vi "testV10-AlmostDone.vi"() -> ()   [LabVIEW 2020]
uses:
  <vilib>/DAQmx/read.llb/DAQmx Read (Analog 2D DBL NChan NSamp).vi
  <vilib>/Analysis/baseanly.llb/Mean (DBL).vi
  <vilib>/DAQmx/miscellaneous.llb/DAQmx Fill In Error Info.vi
  <vilib>/Analysis/NI_AALBase.lvlib
  <resource>/objmgr/daqmx.rc
panel:
  out "index of Module 3":i32
  out "index of Module 2":i32
  out "double precision float":dbl
  out "Time Stamp":timestamp=timestamp(-21600 s since 1904-01-01)
  out "subarray 2":string[](array[string])
  out "index of Module 1":i32
  out "subarray":string[](array[string])
  in  "Counter":dbl
  out ".not. (x .or. y)?":bool
  out "index of element":i32
  out "element":dbl
  out "?":timestamp
  out "Channels":refnum<k21>[](array[refnum])
  out "size(s)":i32
  out "NumDevices":u32
  out "x/y":dbl
  in  "?":T1(tab)
  out "Sampling Status":bool
  in  "Sampling Time":u32=5
  in  "Read Time (s)":u32=60
  in  "Channel List":string(combo)="Temperature"
  out "Read Count Daily":string="0" caption="Timestamp"
  out "Countdown to Read":string="0\n 6:17:48 PM" caption="Timestamp"
  out "?":string="Timestamp"
  out "?":string="File Location"
  out "Timestamp":string="7/26/2020\n 6:17:48 PM"
  in  "Start":bool
  in  "Next Button":bool
  in  "Stop Button 2":bool
  out "Graph Running":bool
  in  "Resolution":u8=10 min=10
  in  "Stop Button":bool
  in  "Play Button":bool
  out "Module 3":bool
  out "Module 2":bool
  out "Module 1":bool
  out "3":bool
  out "2":bool
  out "1":bool
  in  "Running Module":u8=1 min=1 max=3
  in  "Module 3 Task":refnum<k21>="MyTemperatureTask_2"
  out "?":waveform(dbl)(graph)
  in  "Module 3 File Data Location":path=path "E:/KMUTT/Master Degree/labviewjgsee/log/Module3"
  in  "Module 2 File Data Location":path=path "E:/KMUTT/Master Degree/labviewjgsee/log/Module2"
  in  "Module 2 Task":refnum<k21>="MyTemperatureTask_1"
  in  "Module 1 File Data Location":path=path "E:/KMUTT/Master Degree/labviewjgsee/log/Module1"
  in  "Module 1 Task":refnum<k21>="MyTemperatureTask"
  in  "DAQmx Device Name":tag="JGSEE"
  out "Table Module 1":string[][](table)
  out "Table Module 2":string[][](table)
  out "Table Module 3":string[][](table)
  in  "Select Channel Module 1":string(combo)
  out "?":string="Date"
  out "Timestamp 2":string="7/26/2020\n 6:17:48 PM" caption="Timestamp"
  out "Graph Module 1":cluster{timestamp[], dbl[]}[](graph)
  in  "Select Channel Module 2":string(combo)
  out "?":string="Date"
  out "Timestamp 3":string="7/26/2020\n 6:17:48 PM" caption="Timestamp"
  out "Graph Module 2":cluster{timestamp[], dbl[]}[](graph)
  in  "Select Channel Module 3":string(combo)
  out "?":string="Date"
  out "Timestamp 4":string="7/26/2020\n 6:17:48 PM" caption="Timestamp"
  out "Graph Module 3":cluster{timestamp[], dbl[]}[](graph)
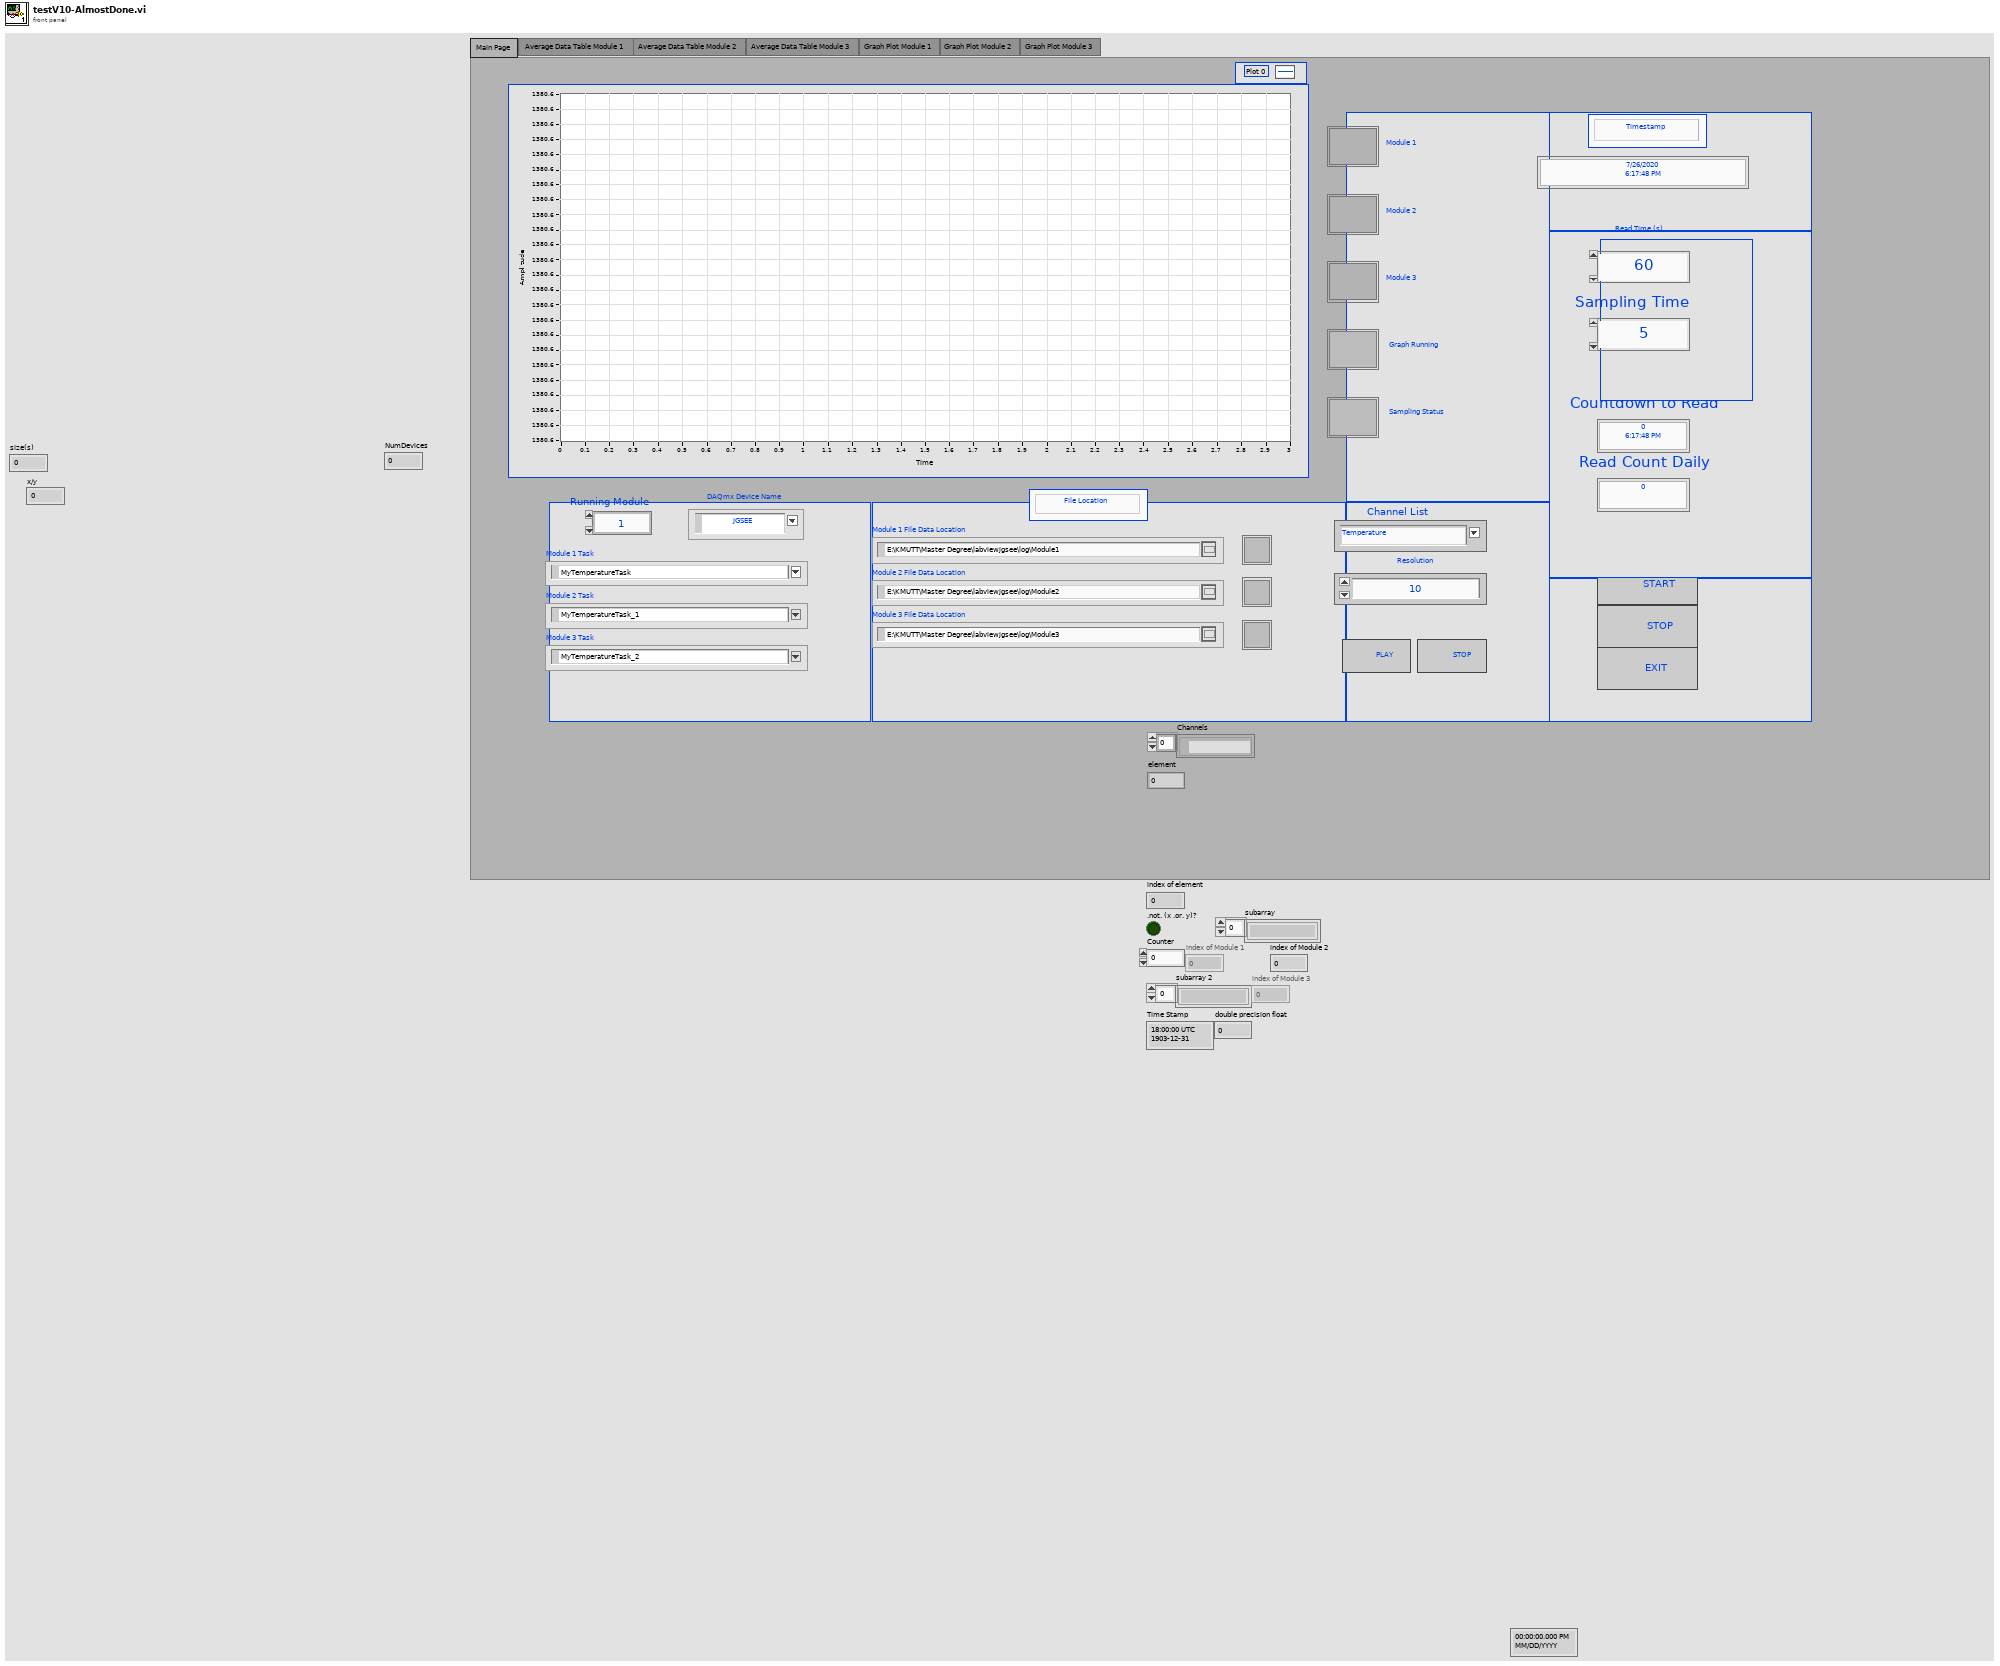
[diagram p1: front panel]
types:
  T1 = enum32{"Main Page ", " Average Data Table Module 1", "Average Data Table Module 2", "Average Data Table Module 3", "Graph Plot Module 1", "Graph Plot Module 2", "Graph Plot Module 3"}
  T2 = enum16{"open", "replace", "create", "open or create", "replace or create", "replace or create with confirmation"}
  T3 = enum8{"Enabled", "Disabled", "Disabled and Grayed Out"}
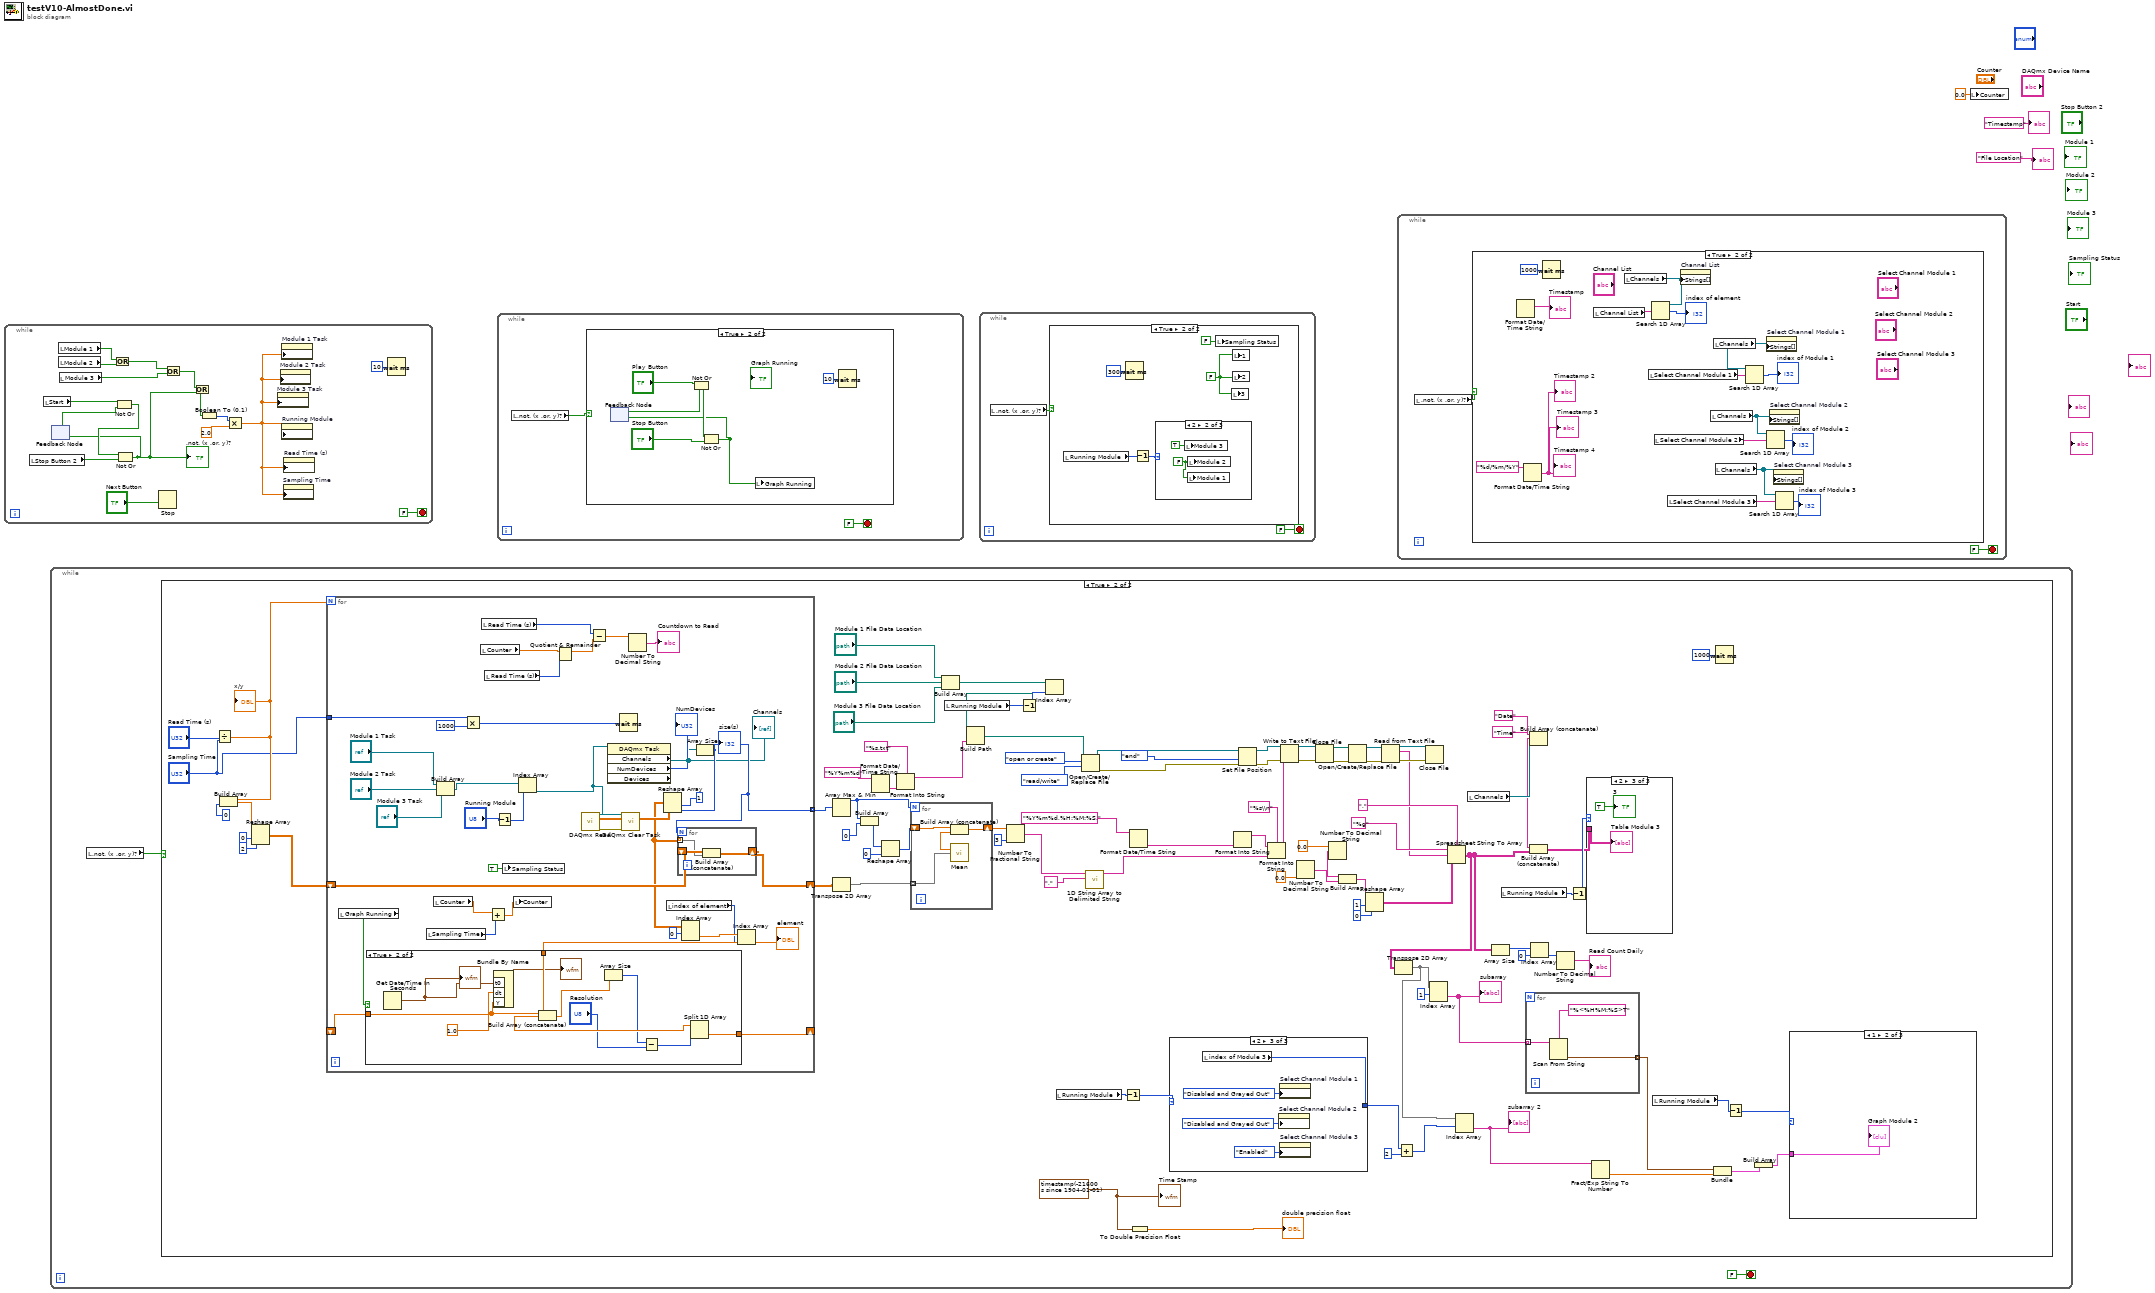
[diagram p0: block diagram]
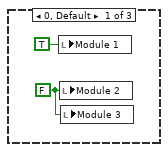
[diagram p4: hidden frame]
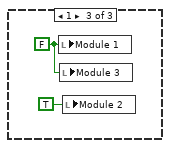
[diagram p5: hidden frame]
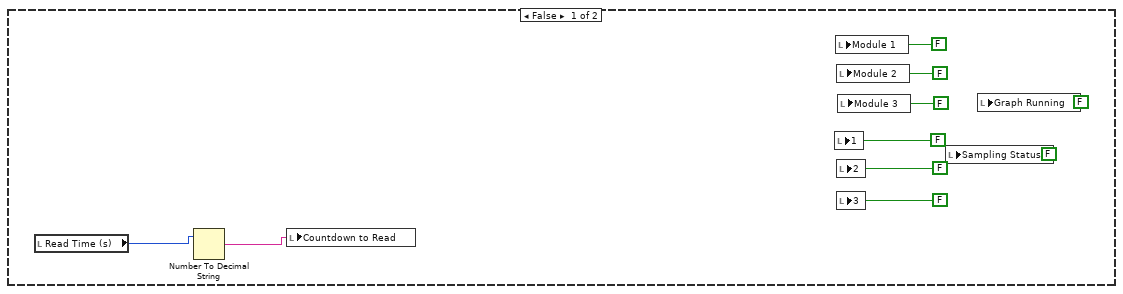
[diagram p7: hidden frame]
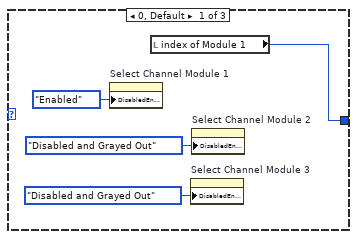
[diagram p8: hidden frame]
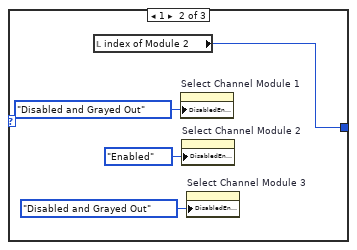
[diagram p9: hidden frame]
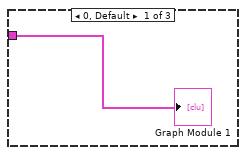
[diagram p10: hidden frame]
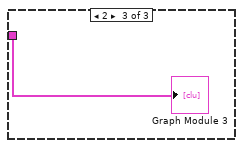
[diagram p11: hidden frame]
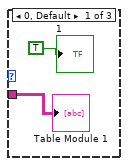
[diagram p12: hidden frame]
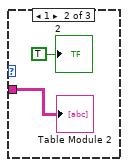
[diagram p13: hidden frame]
diagram:
  n1 = while {
    stop <- FALSE stop-if-true
    n2 = local read "Stop Button 2"() -> (w19:bool)
    n3 = local read "Start"() -> (w14:bool)
    n4 = feedback #1() -> (w17:bool)  [unwired: 1 in]
    n5 = local read "Module 1"() -> (w12:bool)
    n6 = local read "Module 2"() -> (w11:bool)
    n7 = local read "Module 3"() -> (w9:bool)
    n8 = Or(x=w12, y=w11) -> (x .or. y?=w10:bool)
    n9 = Not Or(1:w17, 2:w14) -> (0:w18:bool)
    n10 = Not Or(1:w19, 2:w18) -> (0:w6:bool)
    ".not. (x .or. y)?" <- w6
    n11 = feedback-in #1(w6) -> ()
    n12 = Stop(stop? (T)="Next Button") -> ()
    n13 = Or(x=w10, y=w9) -> (x .or. y?=w8:bool)
    n14 = Or(x=w8, y=w6) -> (x .or. y?=w5:bool)
    n15 = Boolean To (0,1)(Boolean=w5) -> (0, 1=w7:i16)
    n16 = Multiply(x=w7, y=2.0) -> (x*y=w4:dbl)
    n17 = property on="Module 3 Task" class="DAQmxName (strict)"("DisabledEnum"=w4) -> ()  [unwired: 2 in, 2 out]
    n18 = property on="Module 2 Task" class="DAQmxName (strict)"("DisabledEnum"=w4) -> ()  [unwired: 2 in, 2 out]
    n19 = property on="Module 1 Task" class="DAQmxName (strict)"("DisabledEnum"=w4) -> ()  [unwired: 2 in, 2 out]
    n20 = property on="Running Module" class="DigNum (strict)"("DisabledEnum"=w4) -> ()  [unwired: 2 in, 2 out]
    n21 = property on="Sampling Time" class="DigNum (strict)"("DisabledEnum"=w4) -> ()  [unwired: 2 in, 2 out]
    n22 = property on="Read Time (s)" class="DigNum (strict)"("DisabledEnum"=w4) -> ()  [unwired: 2 in, 2 out]
    n23 = Wait (ms)(milliseconds to wait=u32 10) -> ()  [unwired: 1 out]
  }
  n24 = while {
    stop <- FALSE stop-if-true
    n25 = local read ".not. (x .or. y)?"() -> (w21:bool)
    n26 = case shown="True" w21 {
      frame False {
        n27 = local read "Read Time (s)"() -> (w24:u32)
        n28 = Number To Decimal String(number=w24) -> (decimal integer string=w23:string)  [unwired: 1 in]
        n29 = local write "Countdown to Read"(w23) -> ()
        n30 = local write "1"(FALSE ("1")) -> ()
        n31 = local write "Module 1"(FALSE ("Module 1")) -> ()
        n32 = local write "Module 2"(FALSE ("Module 2")) -> ()
        n33 = local write "2"(FALSE ("2")) -> ()
        n34 = local write "3"(FALSE ("3")) -> ()
        n35 = local write "Module 3"(FALSE ("Module 3")) -> ()
        n36 = local write "Sampling Status"(FALSE ("Sampling Status")) -> ()
        n37 = local write "Graph Running"(FALSE ("Graph Running")) -> ()
      }
      frame True {
        w40 = timestamp(-21600 s since 1904-01-01)
        n38 = Divide(x="Read Time (s)", y="Sampling Time") -> (x/y=w102:dbl)
        "x/y" <- w102
        n39 = Build Array(w102, 0 ("element")) -> (w106:dbl[])
        n40 = Reshape Array(w106, 0 ("dimension size"), 2 ("dimension size")) -> (w103:dbl[][])
        n41 = for {
          N: w102 -> [_]
          shift-right: [w184] -> w71
          shift-left: w103 -> [w183]
          tunnel: "Sampling Time" -> [w182]
          tunnel: [w180] -> w101 mode=indexing
          shift-right: [w164] -> _
          shift-left: _ -> [w163]
          n42 = local read "Graph Running"() -> (w162:bool)
          n43 = local read "Sampling Time"() -> (w158:u32)
          n44 = local read "Counter"() -> (w157:dbl)
          n45 = Build Array("Module 1 Task", "Module 2 Task", "Module 3 Task") -> (w175:refnum<k21>[])
          n46 = Multiply(x=w182, y=u32 1000) -> (x*y=w170:u32)
          n47 = local read "Counter"() -> (w151:dbl)
          n48 = local read "Read Time (s)"() -> (w154:u32)
          n49 = local read "Read Time (s)"() -> (w156:u32)
          n50 = Add(x=w157, y=w158) -> (x+y=w159:dbl)
          n51 = Decrement(x="Running Module") -> (x-1=w171:u8)
          n52 = local write "Sampling Status"(TRUE ("Sampling Status")) -> ()
          n53 = local write "Counter"(w159) -> ()
          n54 = Index Array(array=w175, index=w171) -> (element=w174:refnum<k21>)
          n55 = Quotient & Remainder(x=w151, y=w156) -> (x-y*floor(x/y)=w155:dbl)  [unwired: 1 out]
          n56 = call-poly <vilib>:"DAQmx Read.vi"("task/channels in"=w174) -> ("task out"=w186:refnum<k21>, "data"=w179:dbl[][], "error out"=w187:errorcluster)  [unwired: 12 in]
          n57 = Subtract(x=w154, y=w155) -> (x-y=w153:dbl)
          n58 = property class="DAQmx Task" props=["Channels", "NumDevices", "Devices"](reference=w174) -> ("Channels"=w169:refnum<k21>[], "NumDevices"=→"NumDevices":u32)  [unwired: 1 in, 3 out]
          "Channels" <- w169
          n59 = Wait (ms)(milliseconds to wait=w170) -> ()  [unwired: 1 out]
          n60 = call <vilib>:"DAQmx Clear Task.vi"("task in"=w186, "error in"=w187) -> ()  [unwired: 13 in, 1 out]
          n61 = Number To Decimal String(number=w153) -> (decimal integer string=→"Countdown to Read":string)  [unwired: 1 in]
          n62 = local read "index of element"() -> (w161:i32)
          n63 = Array Size(array=w169) -> (size(s)=w180:i32)
          "size(s)" <- w180
          n64 = Reshape Array(w179, 1 ("dimension size"), w180) -> (w168:dbl[][])
          n65 = for {
            N: w180 -> [_]
            shift-right: [w199] -> w184
            shift-left: w183 -> [w200]
            tunnel: w168 -> [w198] mode=indexing
            n66 = Build Array (concatenate)(w200, w198) -> (w199:dbl[][])
          }
          n67 = Index Array(array=w168, index (row)=0) -> (element=w166:dbl[])  [unwired: 1 in]
          n68 = Index Array(array=w166, index=w161) -> (element=w165:dbl)
          "element" <- w165
          n69 = case shown="True" w162 {
            tunnel: w165 -> [_ w195]
            tunnel: [_ w192] -> w164
            tunnel: w163 -> [_ w191]
            frame False {
            }
            frame True {
              n70 = Get Date/Time In Seconds() -> (seconds since 1Jan1904=w197:timestamp)
              "?" <- w197
              n71 = Bundle By Name("t0"=w197, "dt"=1.0, "Y"=w191) -> (→"?":waveform(dbl))  [unwired: 1 in]
              n72 = Build Array (concatenate)(w191, w195) -> (w193:dbl[])
              n73 = Array Size(array=w193) -> (size(s)=w189:i32)
              n74 = Subtract(x=w189, y="Resolution") -> (x-y=w190:i32)
              n75 = Split 1D Array(array=w193, index=w190) -> (second subarray=w192:dbl[])  [unwired: 1 out]
            }
          }
        }
        n76 = Array Max & Min(array=w101) -> (max value=w98:i32)  [unwired: 3 out]
        n77 = Transpose 2D Array(2D array=w71) -> (transposed array=w100:dbl[][])
        n78 = Build Array(w98, 0 ("element")) -> (w96:i32[])
        n79 = Format Date/Time String(time format string (%c)="%Y%m%d") -> (date/time string=w118:string)  [unwired: 2 in]
        n80 = Reshape Array(w96, 0 ("dimension size")) -> (w95:i32[])
        n81 = Format Into String(format string="%s.txt", w118) -> (resulting string=w116:string)  [unwired: 2 in, 1 out]
        n82 = for {
          N: w98 -> [_]
          tunnel: w100 -> [w204] mode=indexing
          shift-right: [w202] -> w108
          shift-left: w95 -> [w201]
          n83 = call-poly <vilib>:"Mean.vi"("X"=w204) -> ("mean"=w203:dbl)  [unwired: 1 out]
          n84 = Build Array (concatenate)(w201, w203) -> (w202:dbl[])
        }
        n85 = Build Array("Module 1 File Data Location", "Module 2 File Data Location", "Module 3 File Data Location") -> (w64:path[])
        n86 = local read "Running Module"() -> (w65:u8)
        n87 = Number To Fractional String(number=w108, precision (6)=i16 3) -> (F-format string=w109:string[])  [unwired: 2 in]
        n88 = Decrement(x=w65) -> (x-1=w63:u8)
        n89 = Index Array(array=w64, index=w63) -> (element=w62:path)
        n90 = Build Path(base path=w62, name or relative path=w116) -> (appended path=w115:path)
        n91 = local read "Running Module"() -> (w38:u8)
        n92 = Open/Create/Replace File(file path (use dialog)=w115, operation (0:open)=T2."open or create", access (0:read/write)=enum16{"read/write", "read-only", "write-only"}."read/write") -> (refnum out=w93:refnum<file>, error out=w122:errorcluster)  [unwired: 3 in, 1 out]
        n93 = call <vilib>:"1D String Array to Delimited String.vi"("delimiter"="," ("format string"), "string array"=w109) -> ("delimited string"=w114:string)  [unwired: 9 in]
        n94 = Decrement(x=w38) -> (x-1=w37:u8)
        n95 = Format Date/Time String(time format string (%c)="%Y%m%d,%H:%M:%S,") -> (date/time string=w111:string)  [unwired: 2 in]
        n96 = To Double Precision Float(number=w40) -> (double precision float=→"double precision float":dbl)
        n97 = case shown="2" w37 {
          tunnel: [w130 w134 w138] -> w33
          frame 0, Default {
            n98 = property on="Select Channel Module 1" class="CmbBox"("DisabledEnum"=T3."Enabled" ("Disabled")) -> ()  [unwired: 2 in, 2 out]
            n99 = local read "index of Module 1"() -> (w130:i32)
            n100 = property on="Select Channel Module 3" class="CmbBox"("DisabledEnum"=T3."Disabled and Grayed Out" ("Disabled")) -> ()  [unwired: 2 in, 2 out]
            n101 = property on="Select Channel Module 2" class="CmbBox"("DisabledEnum"=T3."Disabled and Grayed Out" ("Disabled")) -> ()  [unwired: 2 in, 2 out]
          }
          frame 1 {
            n102 = local read "index of Module 2"() -> (w134:i32)
            n103 = property on="Select Channel Module 1" class="CmbBox"("DisabledEnum"=T3."Disabled and Grayed Out" ("Disabled")) -> ()  [unwired: 2 in, 2 out]
            n104 = property on="Select Channel Module 2" class="CmbBox"("DisabledEnum"=T3."Enabled" ("Disabled")) -> ()  [unwired: 2 in, 2 out]
            n105 = property on="Select Channel Module 3" class="CmbBox"("DisabledEnum"=T3."Disabled and Grayed Out" ("Disabled")) -> ()  [unwired: 2 in, 2 out]
          }
          frame 2 {
            n106 = local read "index of Module 3"() -> (w138:i32)
            n107 = property on="Select Channel Module 2" class="CmbBox"("DisabledEnum"=T3."Disabled and Grayed Out" ("Disabled")) -> ()  [unwired: 2 in, 2 out]
            n108 = property on="Select Channel Module 1" class="CmbBox"("DisabledEnum"=T3."Disabled and Grayed Out" ("Disabled")) -> ()  [unwired: 2 in, 2 out]
            n109 = property on="Select Channel Module 3" class="CmbBox"("DisabledEnum"=T3."Enabled" ("Disabled")) -> ()  [unwired: 2 in, 2 out]
          }
        }
        n110 = Format Into String(w111) -> (resulting string=w110:string)  [unwired: 3 in, 1 out]
        n111 = Set File Position(refnum=w93, from (0:start)=enum16{"start", "end", "current"}."end", error in=w122) -> (refnum out=w123:refnum<file>, error out=w121:errorcluster)  [unwired: 1 in]
        n112 = Format Into String(format string="%s\\n", initial string=w110, w114) -> (resulting string=w85:string)  [unwired: 1 in, 1 out]
        n113 = Write to Text File(file (use dialog)=w123, text=w85, error in=w121) -> (refnum out=w92:refnum<file>, error out=w91:errorcluster)  [unwired: 1 in, 1 out]
        n114 = Number To Decimal String(number=0.0 ("element")) -> (decimal integer string=w73:string)  [unwired: 1 in]
        n115 = Close File(refnum=w92, error in=w91) -> (path=w90:path, error out=w89:errorcluster)
        n116 = Number To Decimal String(number=0.0 ("element")) -> (decimal integer string=w75:string)  [unwired: 1 in]
        n117 = Build Array(w75, w73) -> (w77:string[])
        n118 = Open/Create/Replace File(file path (use dialog)=w90, error in=w89) -> (refnum out=w88:refnum<file>, error out=w87:errorcluster)  [unwired: 4 in, 1 out]
        n119 = Reshape Array(w77, 1 ("dimension size"), 0 ("dimension size")) -> (w78:string[][])
        n120 = Read from Text File(file (use dialog)=w88, error in=w87) -> (refnum out=w86:refnum<file>, text=w81:string, error out=w82:errorcluster)  [unwired: 2 in, 1 out]
        n121 = Add(x=w33, y=2) -> (x+y=w46:i32)
        n122 = Close File(refnum=w86, error in=w82) -> ()  [unwired: 2 out]
        n123 = Spreadsheet String To Array(delimiter (Tab)=",", format string="%g", spreadsheet string=w81, array type (2D Dbl)=w78) -> (array=w50:string[][])
        n124 = Transpose 2D Array(2D array=w50) -> (transposed array=w47:string[][])
        n125 = Index Array(array=w47, index (row)=1 ("index")) -> (element=w45:string[])  [unwired: 1 in]
        "subarray" <- w45
        n126 = Index Array(array=w47, index (row)=w46) -> (element=w43:string[])  [unwired: 1 in]
        "subarray 2" <- w43
        n127 = local read "Channels"() -> (w56:refnum<k21>[])
        n128 = Array Size(array=w50) -> (size(s)=w54:i32[])
        n129 = local read "Running Module"() -> (w61:u8)
        n130 = for {
          tunnel: w45 -> [w143] mode=indexing
          tunnel: [w142] -> w41 mode=indexing
          n131 = Scan From String(format string="%<%H%M:%S>T", input string=w143) -> (output 1=w142:timestamp)  [unwired: 3 in, 3 out]
        }
        n132 = Build Array (concatenate)("Date", "Time", w56) -> (w55:string[])
        n133 = Build Array (concatenate)(w55, w50) -> (w59:string[][])
        n134 = Index Array(array=w54, index=0) -> (element=w52:i32)
        n135 = Number To Decimal String(number=w52) -> (decimal integer string=→"Read Count Daily":string)  [unwired: 1 in]
        n136 = Decrement(x=w61) -> (x-1=w60:u8)
        n137 = case shown="2" w60 {
          tunnel: w59 -> [w146 w148 w150]
          frame 0, Default {
            "Table Module 1" <- w146
            "1" <- TRUE ("1")
          }
          frame 1 {
            "Table Module 2" <- w148
            "2" <- TRUE ("2")
          }
          frame 2 {
            "Table Module 3" <- w150
            "3" <- TRUE ("3")
          }
        }
        n138 = Fract/Exp String To Number(string=w43) -> (number=w42:dbl[])  [unwired: 3 in, 1 out]
        n139 = local read "Running Module"() -> (w36:u8)
        n140 = Bundle(w41, w42) -> (w44:cluster{timestamp[], dbl[]})  [unwired: 1 in]
        n141 = Wait (ms)(milliseconds to wait=u32 1000) -> ()  [unwired: 1 out]
        n142 = Decrement(x=w36) -> (x-1=w35:u8)
        n143 = Build Array(w44) -> (w34:cluster{timestamp[], dbl[]}[])
        n144 = case shown="1" w35 {
          tunnel: w34 -> [w139 w140 w141]
          frame 0, Default {
            "Graph Module 1" <- w139
          }
          frame 1 {
            "Graph Module 2" <- w140
          }
          frame 2 {
            "Graph Module 3" <- w141
          }
        }
        "Time Stamp" <- w40
      }
    }
  }
  n145 = while {
    stop <- FALSE stop-if-true
    n146 = local read ".not. (x .or. y)?"() -> (w205:bool)
    n147 = case shown="True" w205 {
      frame False {
      }
      frame True {
        n148 = feedback #2() -> (w208:bool)  [unwired: 1 in]
        n149 = Not Or(1:w208, 2:"Play Button") -> (0:w209:bool)
        n150 = Not Or(1:"Stop Button", 2:w209) -> (0:w207:bool)
        n151 = feedback-in #2(w207) -> ()
        n152 = local write "Graph Running"(w207) -> ()
        n153 = Wait (ms)(milliseconds to wait=u32 10) -> ()  [unwired: 1 out]
      }
    }
  }
  n154 = while {
    stop <- FALSE stop-if-true
    n155 = local read ".not. (x .or. y)?"() -> (w213:bool)
    n156 = case shown="True" w213 {
      frame False {
      }
      frame True {
        w218 = FALSE ("1")
        n157 = local read "Running Module"() -> (w216:u8)
        n158 = Wait (ms)(milliseconds to wait=u32 300) -> ()  [unwired: 1 out]
        n159 = Decrement(x=w216) -> (x-1=w215:u8)
        n160 = case shown="2" w215 {
          frame 0, Default {
            w221 = FALSE ("Module 2")
            n161 = local write "Module 1"(TRUE ("Module 1")) -> ()
            n162 = local write "Module 2"(w221) -> ()
            n163 = local write "Module 3"(w221) -> ()
          }
          frame 2 {
            w223 = FALSE ("Module 2")
            n164 = local write "Module 3"(TRUE ("Module 3")) -> ()
            n165 = local write "Module 1"(w223) -> ()
            n166 = local write "Module 2"(w223) -> ()
          }
          frame 1 {
            w225 = FALSE ("Module 1")
            n167 = local write "Module 1"(w225) -> ()
            n168 = local write "Module 3"(w225) -> ()
            n169 = local write "Module 2"(TRUE ("Module 2")) -> ()
          }
        }
        n170 = local write "Sampling Status"(FALSE ("Sampling Status")) -> ()
        n171 = local write "3"(w218) -> ()
        n172 = local write "1"(w218) -> ()
        n173 = local write "2"(w218) -> ()
      }
    }
  }
  n174 = while {
    stop <- FALSE stop-if-true
    n175 = local read ".not. (x .or. y)?"() -> (w226:bool)
    n176 = case shown="True" w226 {
      frame False {
      }
      frame True {
        n177 = Format Date/Time String() -> (date/time string=→"Timestamp":string)  [unwired: 3 in]
        n178 = Format Date/Time String(time format string (%c)="%d/%m/%Y") -> (date/time string=→"Timestamp 2" →"Timestamp 3" →"Timestamp 4":string)  [unwired: 2 in]
        n179 = Wait (ms)(milliseconds to wait=u32 1000) -> ()  [unwired: 1 out]
        n180 = local read "Channel List"() -> (w242:string)
        n181 = local read "Channels"() -> (w243:refnum<k21>[])
        n182 = local read "Select Channel Module 1"() -> (w238:string)
        n183 = Search 1D Array(1D array=w243, element=w242) -> (index of element=→"index of element":i32)  [unwired: 1 in]
        n184 = local read "Select Channel Module 2"() -> (w236:string)
        n185 = local read "Select Channel Module 3"() -> (w233:string)
        n186 = property on="Channel List" class="CmbBox"("Strings[]"=w243) -> ()  [unwired: 2 in, 2 out]
        n187 = local read "Channels"() -> (w235:refnum<k21>[])
        n188 = local read "Channels"() -> (w239:refnum<k21>[])
        n189 = local read "Channels"() -> (w232:refnum<k21>[])
        n190 = Search 1D Array(1D array=w239, element=w238) -> (index of element=→"index of Module 1":i32)  [unwired: 1 in]
        n191 = Search 1D Array(1D array=w235, element=w236) -> (index of element=→"index of Module 2":i32)  [unwired: 1 in]
        n192 = property on="Select Channel Module 1" class="CmbBox"("Strings[]"=w239) -> ()  [unwired: 2 in, 2 out]
        n193 = property on="Select Channel Module 2" class="CmbBox"("Strings[]"=w235) -> ()  [unwired: 2 in, 2 out]
        n194 = property on="Select Channel Module 3" class="CmbBox"("Strings[]"=w232) -> ()  [unwired: 2 in, 2 out]
        n195 = Search 1D Array(1D array=w232, element=w233) -> (index of element=→"index of Module 3":i32)  [unwired: 1 in]
      }
    }
  }
  n196 = local write "Counter"(0.0 ("Counter")) -> ()
  "?" <- "File Location" ("String")
  "?" <- "Timestamp"
